vi "Global Cramer Range.vi"(11 "Cramer Range In":dbl) -> (2 "Std":dbl, 3 "Average Cramer Range":dbl)   [LabVIEW 2014]
uses:
  <vilib>/Analysis/NI_AALBase.lvlib
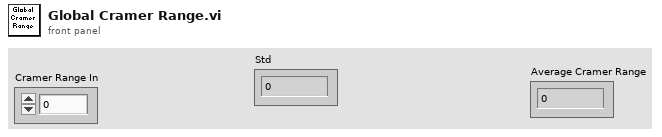
[diagram p1: front panel]
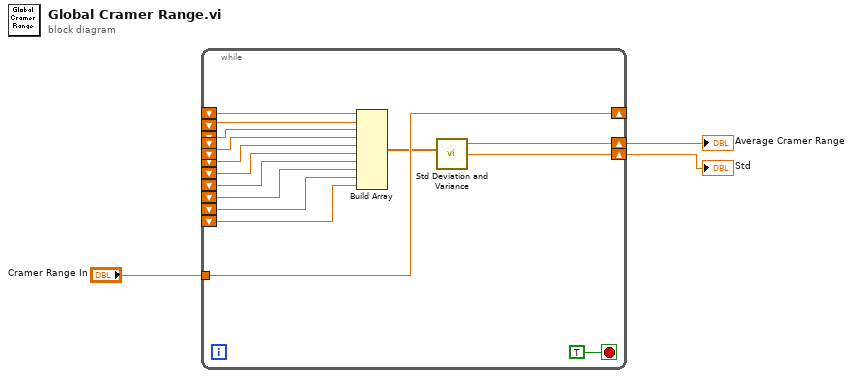
[diagram p0: block diagram]
diagram:
  n1 = while {
    tunnel: "Cramer Range In" -> [w18]
    shift-right: [w18] -> _
    shift-left: _ -> [w12]
    shift-left: _ -> [w13]
    shift-left: _ -> [w14]
    shift-left: _ -> [w15]
    shift-left: _ -> [w16]
    shift-left: _ -> [w17]
    shift-left: _ -> [w11]
    shift-left: _ -> [w10]
    shift-left: _ -> [w9]
    shift-left: _ -> [w8]
    shift-right: [w6] -> w2
    shift-left: _ -> [_]
    shift-right: [w5] -> w1
    shift-left: _ -> [_]
    stop <- TRUE stop-if-true
    n2 = Build Array(w17, w16, w15, w14, w13, w12, w11, w10, w9, w8) -> (w7:dbl[])
    n3 = call <vilib>:"Std Deviation and Variance.vi"("X"=w7) -> ("mean"=w6:dbl, "standard deviation"=w5:dbl)  [unwired: 1 in, 1 out]
  }
  "Average Cramer Range" <- w2
  "Std" <- w1
